vi "AuxLockProb.vi"(7 "CompCoilRef":refnum<vi>, 8 "error in":errorcluster, 9 "Completed loops in":u32, 11 "prob in":dbl) -> (0 "error out":errorcluster, 1 "Completed loops out":u32, 3 "probe lock bools":T2)   [LabVIEW 2019]
uses:
  controls/CompCoilControl.ctl
panel:
  in  "Cluster":T1
  out "output str":string
  # "Current lock :"
  # "Unlock if :"
  # "Probability lock :"
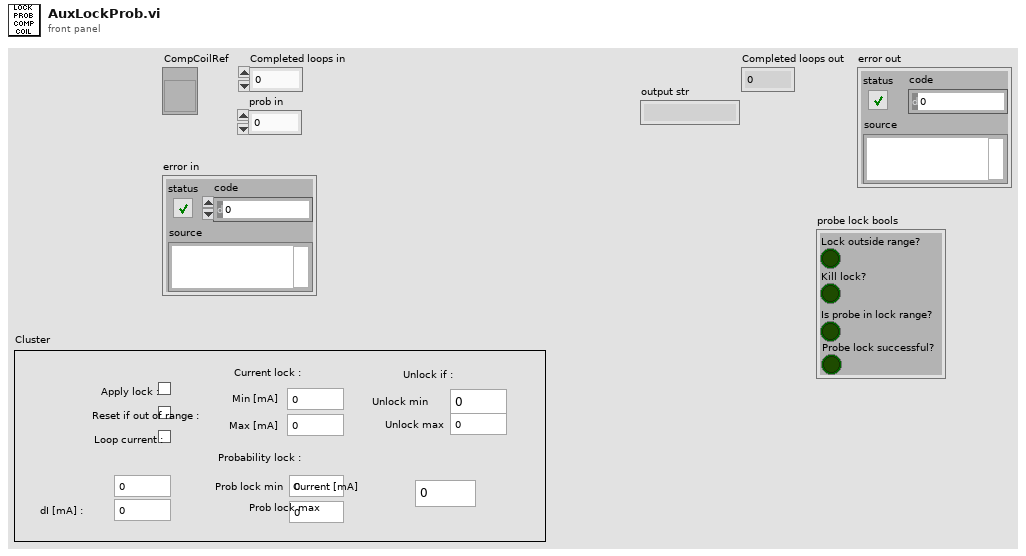
[diagram p1: front panel]
types:
  T1 = typedef "CompCoilControl.ctl" = cluster{"Min [mA]":dbl, "Max [mA]":dbl, "Apply lock :":bool, "Unlock min":dbl, "Unlock max":dbl, "Loop current :":bool, "Reset if out of range :":bool, "Aux runs :":i32, "dI [mA] :":dbl, "Prob lock min ":dbl, "Prob lock max":dbl, "Current [mA]":dbl}
  T2 = cluster{"Lock outside range?":bool, "Kill lock?":bool, "Is probe in lock range?":bool, "Probe lock successful?":bool}
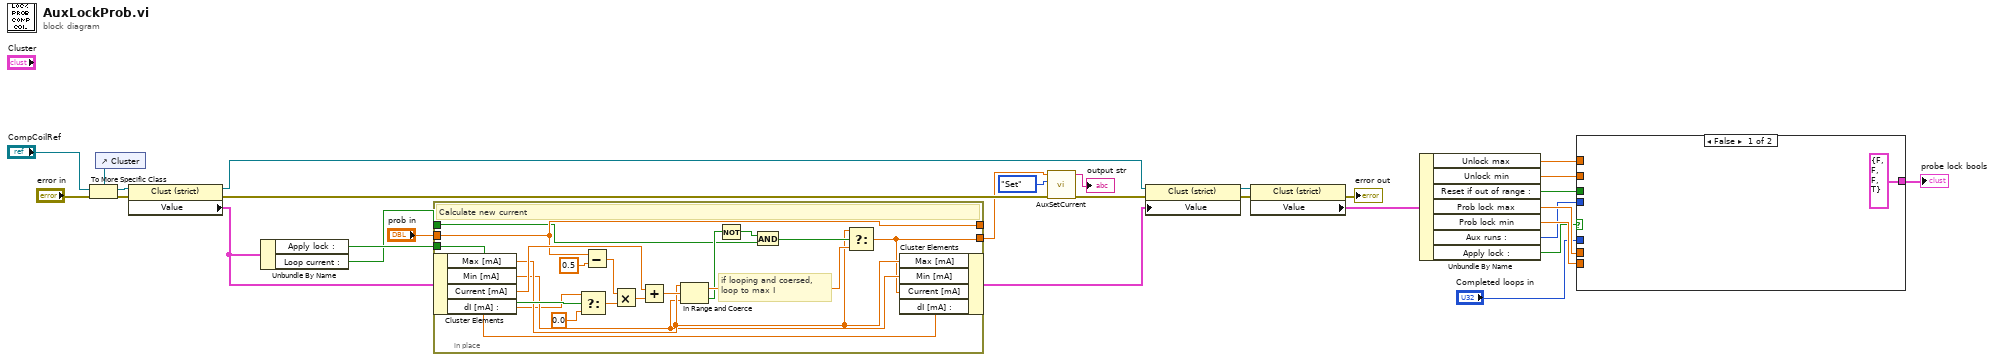
[diagram p0: block diagram]
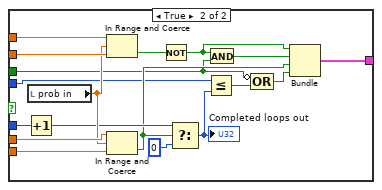
[diagram p2: hidden frame]
diagram:
  n1 = control-ref of="Cluster"() -> (w25:refnum<vi>)
  n2 = To More Specific Class(target class=w25, reference="CompCoilRef", error in="error in") -> (specific class reference=w26:refnum<vi>, error out=w24:errorcluster)
  n3 = property class="Clust (strict)"(reference=w26, error in=w24) -> (reference out=w20:refnum<vi>, error out=w22:errorcluster, "Value"=w14:T1)
  n4 = Unbundle By Name(w14) -> ("Apply lock :"=w13:bool, "Loop current :"=w12:bool)
  n5 = in-place {
    in-place-border: [w36] -> _
    in-place-border: "prob in" -> [w36]
    in-place-border: w12 -> [w35]
    in-place-border: w13 -> [w34]
    in-place-border: [w30] -> w17
    # "if looping and coersed,\nloop to max I"
    # "Calculate new current"
    n6 = in-place-cluster #1(w14) -> ("Max [mA]"=w33:dbl, "Min [mA]"=w32:dbl, "Current [mA]"=w37:dbl, "dI [mA] :"=w31:dbl)
    n7 = Select(t=w31, s=w34, f=0.0) -> (s? t:f=w41:dbl)
    n8 = Subtract(x=w36, y=0.5) -> (x-y=w39:dbl)
    n9 = Multiply(x=w39, y=w41) -> (x*y=w40:dbl)
    n10 = Add(x=w37, y=w40) -> (x+y=w43:dbl)
    n11 = In Range and Coerce(upper limit=w33, x=w43, lower limit=w32) -> (coerced(x)=w47:dbl, In Range?=w44:bool)
    n12 = Not(x=w44) -> (.not. x?=w45:bool)
    n13 = And(x=w45, y=w35) -> (x .and. y?=w46:bool)
    n14 = Select(t=w33, s=w46, f=w47) -> (s? t:f=w30:dbl)
    n15 = in-place-cluster #1("Max [mA]"=w33, "Min [mA]"=w32, "Current [mA]"=w30, "dI [mA] :"=w31) -> (w18:T1)
  }
  n16 = call "AuxSetCurrent.vi"("error in"=w22, "Function select"=enum16{"Init", "Set", "Close"}."Set", "current /mA"=w17) -> ("error out"=w21:errorcluster, "output str"=→"output str":string)  [unwired: 6 in, 1 out]
  n17 = property class="Clust (strict)"(reference=w20, error in=w21, "Value"=w18) -> (reference out=w15:refnum<vi>, error out=w16:errorcluster)
  n18 = property class="Clust (strict)"(reference=w15, error in=w16) -> (error out=→"error out":errorcluster, "Value"=w11:T1)  [unwired: 1 out]
  n19 = Unbundle By Name(w11) -> ("Unlock max"=w10:dbl, "Unlock min"=w9:dbl, "Reset if out of range :"=w4:bool, "Prob lock max"=w8:dbl, "Prob lock min"=w7:dbl, "Aux runs :"=w5:i32, "Apply lock :"=w1:bool)
  n20 = case shown="False" w1 {
    tunnel: w10 -> [_ w66]
    tunnel: w9 -> [_ w65]
    tunnel: w8 -> [_ w64]
    tunnel: w7 -> [_ w63]
    tunnel: "Completed loops in" -> [_ w61]
    tunnel: w5 -> [_ w54]
    tunnel: w4 -> [_ w52]
    tunnel: [cluster{bool, bool, bool, bool} {FALSE, FALSE, FALSE, TRUE} w49] -> w3
    frame False {
    }
    frame True {
      n21 = Increment(x=w61) -> (x+1=w60:u32)
      n22 = local read "prob in"() -> (w62:dbl)
      n23 = In Range and Coerce(upper limit=w66, x=w62, lower limit=w65) -> (In Range?=w58:bool)  [unwired: 1 out]
      n24 = In Range and Coerce(upper limit=w64, x=w62, lower limit=w63) -> (In Range?=w55:bool)  [unwired: 1 out]
      n25 = Not(x=w58) -> (.not. x?=w57:bool)
      n26 = Select(t=w60, s=w55, f=u32 0) -> (s? t:f=w53:u32)
      "Completed loops out" <- w53
      n27 = Less Or Equal?(x=w54, y=w53) -> (x <= y?=w51:bool)
      n28 = And(x=w57, y=w52) -> (x .and. y?=w56:bool)
      n29 = Compound Arithmetic op=OR(invert w52, w51) -> (w50:bool)
      n30 = Bundle(w57, w56, w55, w50) -> (w49:cluster{bool, bool, bool, bool})  [unwired: 1 in]
    }
  }
  "probe lock bools" <- w3
